vi "switch_curve.vi"(9 "字符串":string, 10 "簇":T23, 11 "配置":T1 {"串口通信UI"."Format" items=["标准帧", "扩展帧"]; "串口通信UI"."Type" items=["数据帧", "远程帧"]; "串口通信UI"."ID" format="0x%x"; "串口通信UI"."Fliter" items=["接收所有类型"=1, "只接收标准帧"=2, "只接收扩展帧"=3]; "串口通信UI"."kBaudRate" items=["5k bps"=1, "10k bps"=2, "20k bps"=3, "40k bps"=4, "50k bps"=5, "80k bps"=6, "100k bps"=7, "125k bps"=8, "200k bps"=9, "250k bps"=10, "400k bps"=11, "500k bps"=12, "666k bps"=13, "800k bps"=14, "1000k bps"=15, "33.33k bps"=16, "66.66k bps"=17, "83.33k bps"=18]; "串口通信UI"."Mode" items=["正常工作", "仅侦听模式", "自测模式（环回）"]; "串口通信UI"."InitFlag" items=["使用界面设置参数"=1]; "串口通信UI"."AccMask" format="%08x"; "串口通信UI"."AccCode" format="%08x"; "串口通信UI"."Channel" items=["通道1", "通道2"]; "串口通信UI"."DevType" items=["USB-CAN"=3, "USB-CAN2"=4]; "安全报警UI"."操作 8" items=["产生报警信息（不发声），等待手动操作", "产生报警信息（发声），等待手动操作", "产生报警信息（不发声），自动刹车", "产生报警信息（发声），自动刹车", "产生报警信息（不发声），立即自动断电，开启泄放电阻", "产生报警信息（发声），立即自动断电，开启泄放电阻"]; "安全报警UI"."操作 7" items=["产生报警信息（不发声），等待手动操作", "产生报警信息（发声），等待手动操作", "产生报警信息（不发声），自动刹车", "产生报警信息（发声），自动刹车", "产生报警信息（不发声），立即自动断电，开启泄放电阻", "产生报警信息（发声），立即自动断电，开启泄放电阻"]; "安全报警UI"."操作 6" items=["产生报警信息（不发声），等待手动操作", "产生报警信息（发声），等待手动操作", "产生报警信息（不发声），自动刹车", "产生报警信息（发声），自动刹车", "产生报警信息（不发声），立即自动断电，开启泄放电阻", "产生报警信息（发声），立即自动断电，开启泄放电阻"]; "安全报警UI"."操作 5" items=["产生报警信息（不发声），等待手动操作", "产生报警信息（发声），等待手动操作", "产生报警信息（不发声），自动刹车", "产生报警信息（发声），自动刹车", "产生报警信息（不发声），立即自动断电，开启泄放电阻", "产生报警信息（发声），立即自动断电，开启泄放电阻"]; "安全报警UI"."操作 4" items=["产生报警信息（不发声），等待手动操作", "产生报警信息（发声），等待手动操作", "产生报警信息（不发声），自动刹车", "产生报警信息（发声），自动刹车", "产生报警信息（不发声），立即自动断电，开启泄放电阻", "产生报警信息（发声），立即自动断电，开启泄放电阻"]; "安全报警UI"."操作 3" items=["产生报警信息（不发声），等待手动操作", "产生报警信息（发声），等待手动操作", "产生报警信息（不发声），自动刹车", "产生报警信息（发声），自动刹车", "产生报警信息（不发声），立即自动断电，开启泄放电阻", "产生报警信息（发声），立即自动断电，开启泄放电阻"]; "安全报警UI"."操作 2" items=["产生报警信息（不发声），等待手动操作", "产生报警信息（发声），等待手动操作", "产生报警信息（不发声），自动刹车", "产生报警信息（发声），自动刹车", "产生报警信息（不发声），立即自动断电，开启泄放电阻", "产生报警信息（发声），立即自动断电，开启泄放电阻"]; "安全报警UI"."操作" items=["产生报警信息（不发声），等待手动操作", "产生报警信息（发声），等待手动操作", "产生报警信息（不发声），自动刹车", "产生报警信息（发声），自动刹车", "产生报警信息（不发声），立即自动断电，开启泄放电阻", "产生报警信息（发声），立即自动断电，开启泄放电阻"]}) -> (3 "配置输出":T1 {"串口通信UI"."Format" items=["标准帧", "扩展帧"]; "串口通信UI"."Type" items=["数据帧", "远程帧"]; "串口通信UI"."ID" format="0x%x"; "串口通信UI"."Fliter" items=["接收所有类型"=1, "只接收标准帧"=2, "只接收扩展帧"=3]; "串口通信UI"."kBaudRate" items=["5k bps"=1, "10k bps"=2, "20k bps"=3, "40k bps"=4, "50k bps"=5, "80k bps"=6, "100k bps"=7, "125k bps"=8, "200k bps"=9, "250k bps"=10, "400k bps"=11, "500k bps"=12, "666k bps"=13, "800k bps"=14, "1000k bps"=15, "33.33k bps"=16, "66.66k bps"=17, "83.33k bps"=18]; "串口通信UI"."Mode" items=["正常工作", "仅侦听模式", "自测模式（环回）"]; "串口通信UI"."InitFlag" items=["使用界面设置参数"=1]; "串口通信UI"."AccMask" format="%08x"; "串口通信UI"."AccCode" format="%08x"; "串口通信UI"."Channel" items=["通道1", "通道2"]; "串口通信UI"."DevType" items=["USB-CAN"=3, "USB-CAN2"=4]; "安全报警UI"."操作 8" items=["产生报警信息（不发声），等待手动操作", "产生报警信息（发声），等待手动操作", "产生报警信息（不发声），自动刹车", "产生报警信息（发声），自动刹车", "产生报警信息（不发声），立即自动断电，开启泄放电阻", "产生报警信息（发声），立即自动断电，开启泄放电阻"]; "安全报警UI"."操作 7" items=["产生报警信息（不发声），等待手动操作", "产生报警信息（发声），等待手动操作", "产生报警信息（不发声），自动刹车", "产生报警信息（发声），自动刹车", "产生报警信息（不发声），立即自动断电，开启泄放电阻", "产生报警信息（发声），立即自动断电，开启泄放电阻"]; "安全报警UI"."操作 6" items=["产生报警信息（不发声），等待手动操作", "产生报警信息（发声），等待手动操作", "产生报警信息（不发声），自动刹车", "产生报警信息（发声），自动刹车", "产生报警信息（不发声），立即自动断电，开启泄放电阻", "产生报警信息（发声），立即自动断电，开启泄放电阻"]; "安全报警UI"."操作 5" items=["产生报警信息（不发声），等待手动操作", "产生报警信息（发声），等待手动操作", "产生报警信息（不发声），自动刹车", "产生报警信息（发声），自动刹车", "产生报警信息（不发声），立即自动断电，开启泄放电阻", "产生报警信息（发声），立即自动断电，开启泄放电阻"]; "安全报警UI"."操作 4" items=["产生报警信息（不发声），等待手动操作", "产生报警信息（发声），等待手动操作", "产生报警信息（不发声），自动刹车", "产生报警信息（发声），自动刹车", "产生报警信息（不发声），立即自动断电，开启泄放电阻", "产生报警信息（发声），立即自动断电，开启泄放电阻"]; "安全报警UI"."操作 3" items=["产生报警信息（不发声），等待手动操作", "产生报警信息（发声），等待手动操作", "产生报警信息（不发声），自动刹车", "产生报警信息（发声），自动刹车", "产生报警信息（不发声），立即自动断电，开启泄放电阻", "产生报警信息（发声），立即自动断电，开启泄放电阻"]; "安全报警UI"."操作 2" items=["产生报警信息（不发声），等待手动操作", "产生报警信息（发声），等待手动操作", "产生报警信息（不发声），自动刹车", "产生报警信息（发声），自动刹车", "产生报警信息（不发声），立即自动断电，开启泄放电阻", "产生报警信息（发声），立即自动断电，开启泄放电阻"]; "安全报警UI"."操作" items=["产生报警信息（不发声），等待手动操作", "产生报警信息（发声），等待手动操作", "产生报警信息（不发声），自动刹车", "产生报警信息（发声），自动刹车", "产生报警信息（不发声），立即自动断电，开启泄放电阻", "产生报警信息（发声），立即自动断电，开启泄放电阻"]})   [LabVIEW 2018, in "UI.lvlib"]
uses:
  UI.lvlib
  Settings/Settings.ctl
  Acquisition/Hardware Configuration.ctl
  Acquisition/Signal Type.ctl
  Logging/Logging Configuration.ctl
  Logging/Logging.lvlib
  Acquisition/Acquisition.lvlib
  Settings/Settings.lvlib
panel:
  # "参数配置文件"
  # "输入数据文件"
  # "加载电机"
  # "负载电机"
  # "注：每次运行实验时销毁现有所有图像"
  # "参数配置文件"
  # "输入数据文件"
  # "加载电机"
  # "负载电机"
  # "注：每次运行实验时销毁现有所有图像"
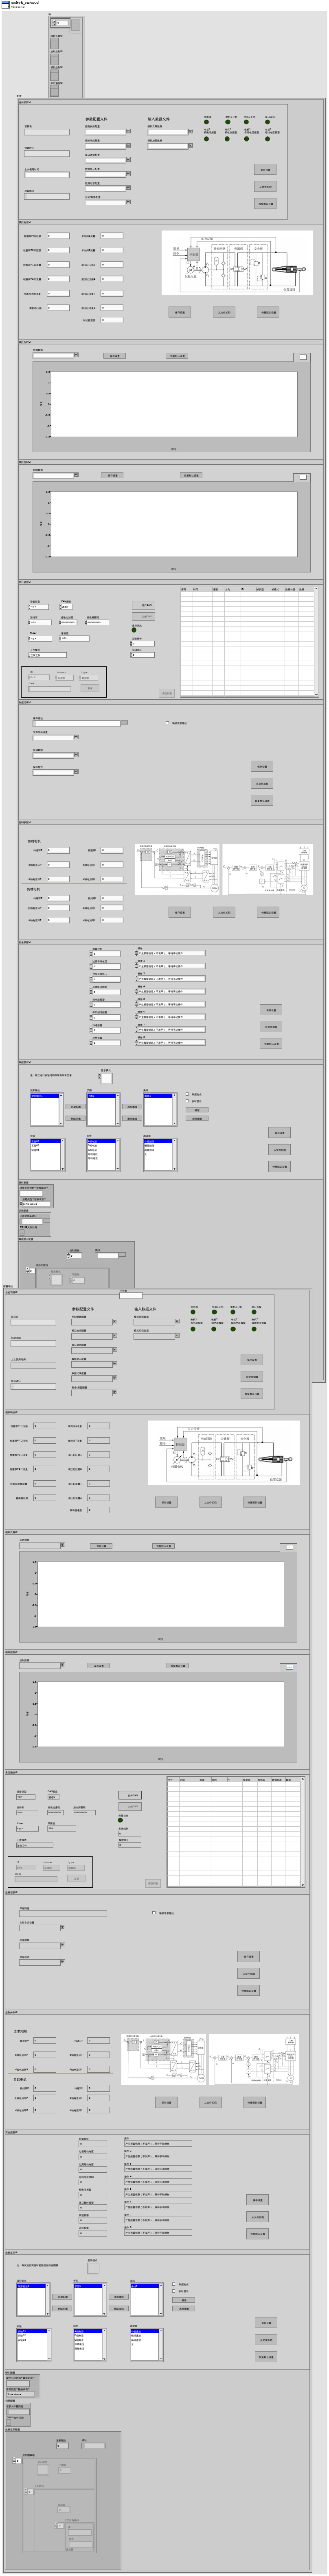
[diagram p1: front panel]
types:
  T1 = typedef "Settings.lvlib/Settings.ctl" = cluster{"当前项目UI":T2, "模拟响应UI":T3, "模拟负载UI":T4, "模拟控制UI":T5, "串口通信UI":T6, "数据记录UI":T12, "控制参数UI":T13, "安全报警UI":T14, "数据显示UI":T15, "硬件配置":T16, "记录配置":T18, "数据显示配置":T19}
  T2 = typedef "控件 5.ctl" = cluster{"控制参数配置":string, "模拟响应配置":string, "串口通信配置":string, "数据显示配置":string, "数据记录配置":string, "安全/报警配置":string, "模拟负载数据":string, "模拟加载数据":string, "总电源":bool, "电机1上电":bool, "电机2上电":bool, "串口连接":bool, "电机1\n相电流报警":bool, "电机2\n相电流报警":bool, "电机1\n母线电压报警":bool, "电机2\n母线电压报警":bool, "保存设置":bool, "从文件加载":bool, "恢复默认设置":bool, "路径":path, "项目路径":path, "项目名":string, "创建时间":string, "上次使用时间":string}
  T3 = typedef "模拟响应UI.ctl" = cluster{"柱塞泵P!口压强":dbl, "柱塞泵P2口压强":dbl, "柱塞泵P1口流量":dbl, "柱塞泵P2口流量":dbl, "柱塞泵泄露流量":dbl, "蓄能器压强":dbl, "单向阀1流量":dbl, "单向阀2流量":dbl, "液压缸压强1":dbl, "液压缸压强2":dbl, "液压缸流量1":dbl, "液压缸流量2":dbl, "做动器速度":dbl, "保存设置":bool, "从文件加载":bool, "恢复默认设置":bool, "路径":path}
  T4 = typedef "控件 9.ctl" = cluster{"负载数据":string, "负载数据 2":waveform(dbl)[], "保存设置":bool, "恢复默认设置":bool}
  T5 = typedef "控件 7.ctl" = cluster{"控制数据":string, "负载数据 2":waveform(dbl)[], "保存设置":bool, "恢复默认设置":bool}
  T6 = typedef "控件 6.ctl" = cluster{"DevType":T7, "Channel":T8, "AccCode":u32, "AccMask":u32, "InitFlag":T9, "Mode":T10, "kBaudRate":u8, "Fliter":T11, "Open":bool, "Close":bool, "连接状态":bool, "SendCnt":u32, "RecvCnt":u32, "Send":bool, "ID":u32, "Data":string, "Type":u8, "Format":u8, "Clear":bool, "list":i32, "路径":path}
  T7 = typedef "ControlCAN.lvlib/DevType.ctl" = u32
  T8 = typedef "ControlCAN.lvlib/CAN Channel.ctl" = u32
  T9 = typedef "ControlCAN.lvlib/InitFlag.ctl" = u32
  T10 = typedef "ControlCAN.lvlib/Mode.ctl" = u8
  T11 = typedef "ControlCAN.lvlib/Fliter.ctl" = u8
  T12 = typedef "控件 3.ctl" = cluster{"保存路径":path, "文件命名设置":string, "存储数据":string, "保存格式":string, "复选框":bool, "保存设置":bool, "从文件加载":bool, "恢复默认设置":bool, "路径":path}
  T13 = typedef "控件 1.ctl" = cluster{"d轴电流环P":dbl, "转速环P":dbl, "q轴电流环P":dbl, "d轴电流环P":dbl, "转矩环P":dbl, "去轴电流环P":dbl, "转速环I":dbl, "q轴电流环I":dbl, "d轴电流环I":dbl, "转矩环I":dbl, "q轴电流环I":dbl, "d轴电流环I":dbl, "保存设置":bool, "从文件加载":bool, "恢复默认设置":bool, "路径":path}
  T14 = typedef "控件 4.ctl" = cluster{"报警扭矩":dbl, "过低母线电压":dbl, "过高母线电压":dbl, "母线电流限制":dbl, "相电流报警":dbl, "串口超时报警":dbl, "转速报警":dbl, "过热报警":dbl, "操作":u16, "操作 2":u16, "操作 3":u16, "操作 4":u16, "操作 5":u16, "操作 6":u16, "操作 7":u16, "操作 8":u16, "保存设置":bool, "从文件加载":bool, "恢复默认设置":bool, "路径":path}
  T15 = typedef "控件 2.ctl" = cluster{"保存设置":bool, "从文件加载":bool, "恢复默认设置":bool, "实验":i32, "波形输出":i32, "组件":i32, "曲线":i32, "滤波器":i32, "删除曲线":bool, "清理图像":bool, "添加曲线":bool, "数据选点":bool, "确定按钮":bool, "实时显示":bool, "子图":i32, "显示模式":u16, "路径":path, "删除图像":bool, "创建新图":bool}
  T16 = typedef "Acquisition.lvlib/Hardware Configuration.ctl" = cluster{"硬件引用句柄<替换此项>":string, "信号类型<替换该项>":T17}
  T17 = typedef "Acquisition.lvlib/Signal Type.ctl" = enum16{"Sine Wave", "Square with Noise"}
  T18 = typedef "Logging.lvlib/Logging Configuration.ctl" = cluster{"记录文件基路径":path, "TDMS文件引用":refnum<k34>}
  T19 = typedef "波形图簇.ctl" = cluster{"波形图数":u32, "波形图数组":T20[], "路径":path}
  T20 = typedef "波形图.ctl" = cluster{"显示模式":u16, "子图数":u32, "子图数组":T21[]}
  T21 = typedef "子图.ctl" = cluster{"子图所有曲线":T22[], "曲线数":u32}
  T22 = typedef "曲线簇.ctl" = cluster{"源":string, "组件":string, "滤波器":string}
  T23 = typedef "引用簇.ctl" = cluster{"数组":refnum<vi>[], "模拟负载UI":refnum<vi>, "波形控制UI":refnum<vi>, "模拟控制UI":refnum<vi>, "串口通信UI":refnum<vi>, "当前项目UI":refnum<vi>, "安全报警UI":refnum<vi>, "数据记录UI":refnum<vi>, "数据显示UI":refnum<vi>, "控制参数UI":refnum<vi>, "模拟响应UI":refnum<vi>, "主选项卡UI":refnum<vi>, "项目管理UI":refnum<vi>, "开始":refnum<vi>, "设置":refnum<vi>, "停止":refnum<vi>, "退出":refnum<vi>}
  T24 = enum8{"Enabled", "Disabled", "Disabled and Grayed Out"}
  T25 = typedef "组件常量.ctl" = string[]
  T26 = typedef "滤波器常量.ctl" = string[]
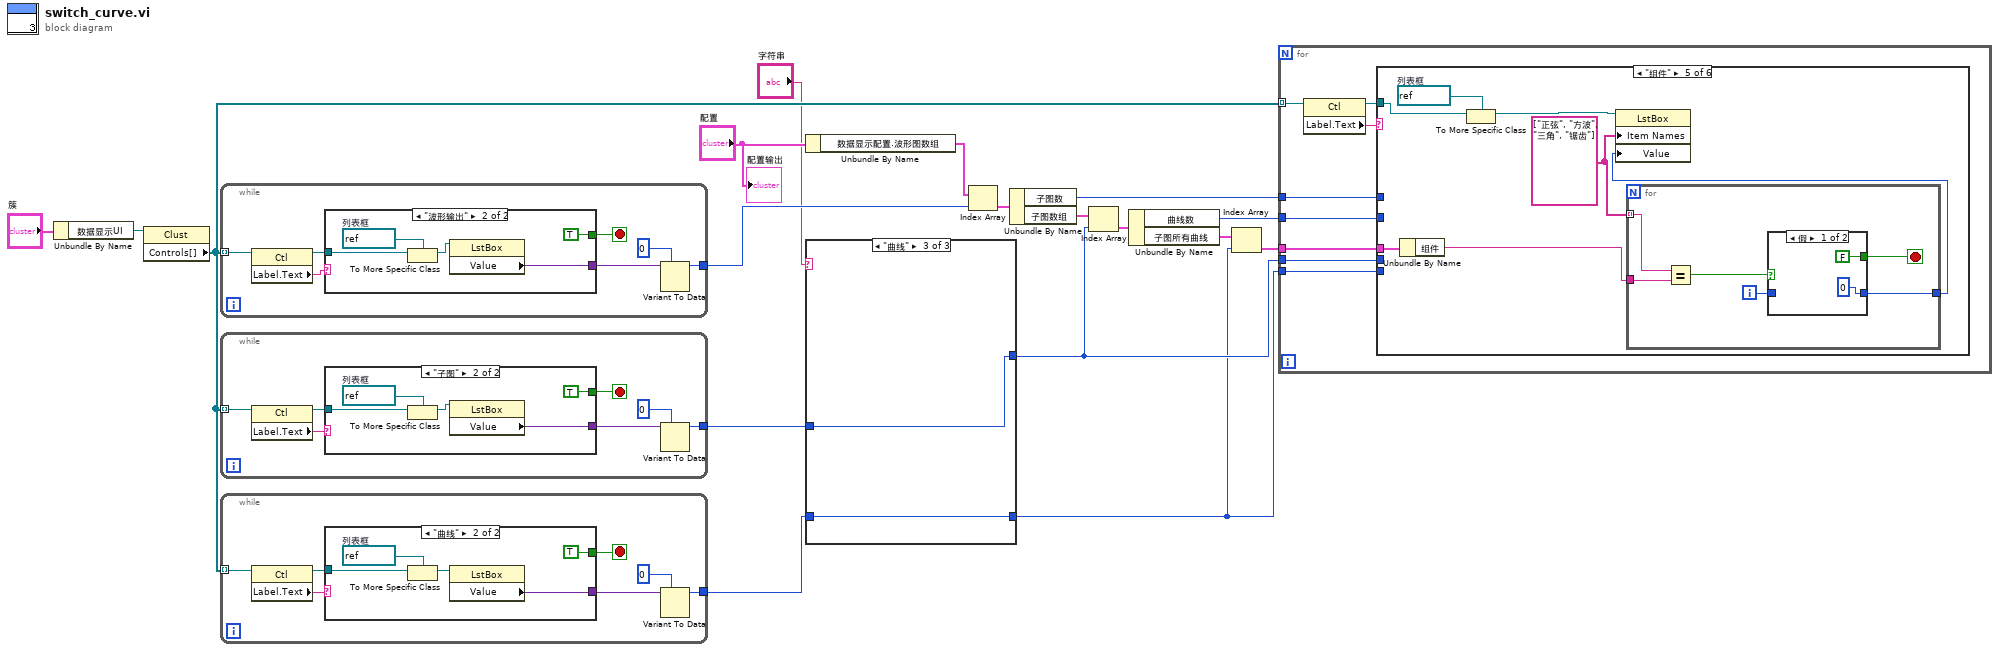
[diagram p0: block diagram]
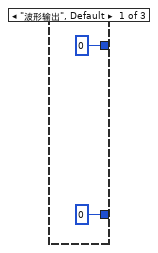
[diagram p2: hidden frame]
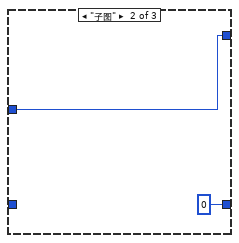
[diagram p3: hidden frame]
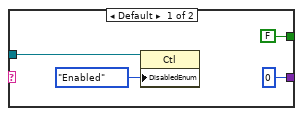
[diagram p4: hidden frame]
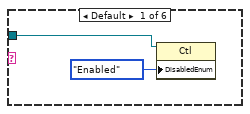
[diagram p5: hidden frame]
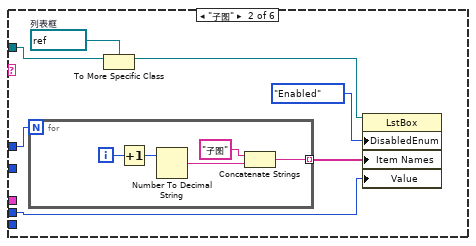
[diagram p6: hidden frame]
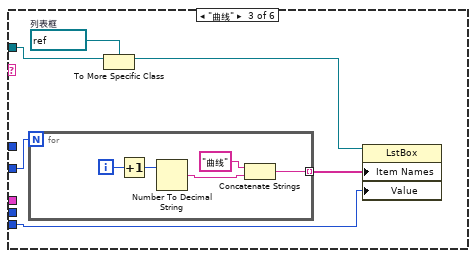
[diagram p7: hidden frame]
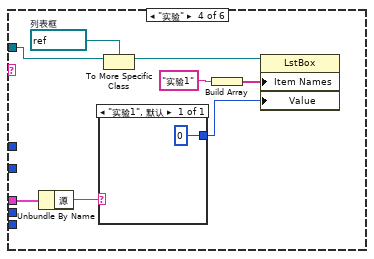
[diagram p8: hidden frame]
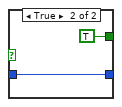
[diagram p9: hidden frame]
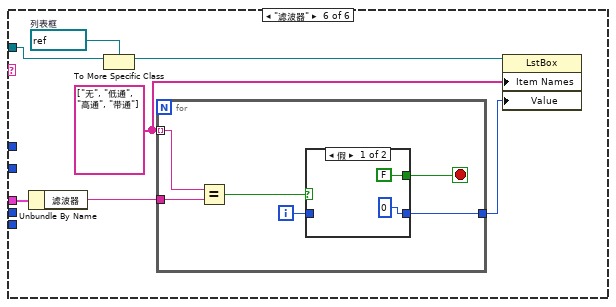
[diagram p10: hidden frame]
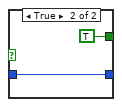
[diagram p11: hidden frame]
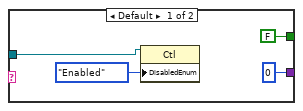
[diagram p12: hidden frame]
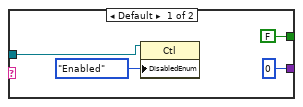
[diagram p13: hidden frame]
diagram:
  n1 = Unbundle By Name("簇") -> ("数据显示UI"=w17:refnum<vi>)
  n2 = property class="Clust"(reference=w17) -> ("Controls[]"=w8:refnum<vi>[])  [unwired: 1 in, 2 out]
  n3 = while {
    tunnel: w8 -> [w25] mode=indexing
    tunnel: [w20] -> w14
    stop <- w22 stop-if-true
    n4 = property class="Ctl"(reference=w25) -> (reference out=w23:refnum<vi>, "Label.Text"=w24:string)  [unwired: 1 in, 1 out]
    n5 = case shown="\"波形输出\"" w24 {
      tunnel: w23 -> [w29 w34]
      tunnel: [0 w30] -> w21
      tunnel: [FALSE TRUE] -> w22
      frame Default {
        n6 = property class="Ctl"(reference=w29, "DisabledEnum"=T24."Enabled" ("禁用")) -> ()  [unwired: 1 in, 2 out]
      }
      frame "波形输出" {
        w33 = refnum<vi> refnum  # 列表框
        n7 = To More Specific Class(target class=w33, reference=w34) -> (specific class reference=w32:refnum<vi>)  [unwired: 1 in, 1 out]
        n8 = property class="LstBox"(reference=w32) -> ("Value"=w30:variant)  [unwired: 1 in, 2 out]
      }
    }
    n9 = Variant To Data(type=0, Variant=w21) -> (data=w20:i32)  [unwired: 1 in, 1 out]
  }
  n10 = while {
    tunnel: w8 -> [w41] mode=indexing
    tunnel: [w36] -> w3
    stop <- w38 stop-if-true
    n11 = property class="Ctl"(reference=w41) -> (reference out=w39:refnum<vi>, "Label.Text"=w40:string)  [unwired: 1 in, 1 out]
    n12 = case shown="\"子图\"" w40 {
      tunnel: w39 -> [w45 w50]
      tunnel: [0 w46] -> w37
      tunnel: [FALSE TRUE] -> w38
      frame Default {
        n13 = property class="Ctl"(reference=w45, "DisabledEnum"=T24."Enabled" ("禁用")) -> ()  [unwired: 1 in, 2 out]
      }
      frame "子图" {
        w49 = refnum<vi> refnum  # 列表框
        n14 = To More Specific Class(target class=w49, reference=w50) -> (specific class reference=w48:refnum<vi>)  [unwired: 1 in, 1 out]
        n15 = property class="LstBox"(reference=w48) -> ("Value"=w46:variant)  [unwired: 1 in, 2 out]
      }
    }
    n16 = Variant To Data(type=0, Variant=w37) -> (data=w36:i32)  [unwired: 1 in, 1 out]
  }
  n17 = while {
    tunnel: w8 -> [w57] mode=indexing
    tunnel: [w52] -> w2
    stop <- w54 stop-if-true
    n18 = property class="Ctl"(reference=w57) -> (reference out=w55:refnum<vi>, "Label.Text"=w56:string)  [unwired: 1 in, 1 out]
    n19 = case shown="\"曲线\"" w56 {
      tunnel: w55 -> [w61 w66]
      tunnel: [0 w62] -> w53
      tunnel: [FALSE TRUE] -> w54
      frame Default {
        n20 = property class="Ctl"(reference=w61, "DisabledEnum"=T24."Enabled" ("禁用")) -> ()  [unwired: 1 in, 2 out]
      }
      frame "曲线" {
        w65 = refnum<vi> refnum  # 列表框
        n21 = To More Specific Class(target class=w65, reference=w66) -> (specific class reference=w64:refnum<vi>)  [unwired: 1 in, 1 out]
        n22 = property class="LstBox"(reference=w64) -> ("Value"=w62:variant)  [unwired: 1 in, 2 out]
      }
    }
    n23 = Variant To Data(type=0, Variant=w53) -> (data=w52:i32)  [unwired: 1 in, 1 out]
  }
  n24 = Unbundle By Name("配置") -> ("数据显示配置.波形图数组"=w15:T20[])
  n25 = case shown="\"曲线\"" "字符串" {
    tunnel: [0 w69 w72] -> w5
    tunnel: [0 0 w71] -> w4
    tunnel: w3 -> [_ w69 w72]
    tunnel: w2 -> [_ _ w71]
    frame "波形输出", Default {
    }
    frame "子图" {
    }
    frame "曲线" {
    }
  }
  n26 = Index Array(array=w15, index=w14) -> (element=w16:T20)
  n27 = Unbundle By Name(w16) -> ("子图数"=w7:u32, "子图数组"=w12:T21[])
  n28 = Index Array(array=w12, index=w5) -> (element=w11:T21)
  n29 = Unbundle By Name(w11) -> ("曲线数"=w1:u32, "子图所有曲线"=w10:T22[])
  n30 = Index Array(array=w10, index=w4) -> (element=w9:T22)
  n31 = for {
    tunnel: w8 -> [w80] mode=indexing
    tunnel: w9 -> [w77]
    tunnel: w4 -> [w76]
    tunnel: w7 -> [w75]
    tunnel: w5 -> [w74]
    tunnel: w1 -> [w73]
    n32 = property class="Ctl"(reference=w80) -> (reference out=w78:refnum<vi>, "Label.Text"=w79:string)  [unwired: 1 in, 1 out]
    n33 = case shown="\"组件\"" w79 {
      tunnel: w78 -> [w82 w85 w96 w113 w121 w138]
      tunnel: w77 -> [_ _ _ w107 w118 w135]
      tunnel: w76 -> [_ _ w100 _ _ _]
      tunnel: w75 -> [_ w84 _ _ _ _]
      tunnel: w74 -> [_ w83 _ _ _ _]
      tunnel: w73 -> [_ _ w95 _ _ _]
      frame Default {
        n34 = property class="Ctl"(reference=w82, "DisabledEnum"=T24."Enabled" ("禁用")) -> ()  [unwired: 1 in, 2 out]
      }
      frame "子图" {
        w88 = refnum<vi> refnum  # 列表框
        n35 = for {
          N: w84 -> [_]
          tunnel: [w92] -> w86 mode=indexing
          i -> [w94]
          n36 = Increment(x=w94) -> (x+1=w90:i32)
          n37 = Number To Decimal String(number=w90) -> (decimal integer string=w91:string)  [unwired: 1 in]
          n38 = Concatenate Strings("子图", w91) -> (w92:string)
        }
        n39 = To More Specific Class(target class=w88, reference=w85) -> (specific class reference=w87:refnum<vi>)  [unwired: 1 in, 1 out]
        n40 = property class="LstBox"(reference=w87, "DisabledEnum"=T24."Enabled" ("禁用"), "Item Names"=w86, "Value"=w83) -> ()  [unwired: 1 in, 2 out]
      }
      frame "曲线" {
        w99 = refnum<vi> refnum  # 列表框
        n41 = for {
          N: w95 -> [_]
          tunnel: [w101] -> w97 mode=indexing
          i -> [w105]
          n42 = Increment(x=w105) -> (x+1=w104:i32)
          n43 = Number To Decimal String(number=w104) -> (decimal integer string=w102:string)  [unwired: 1 in]
          n44 = Concatenate Strings("曲线", w102) -> (w101:string)
        }
        n45 = To More Specific Class(target class=w99, reference=w96) -> (specific class reference=w98:refnum<vi>)  [unwired: 1 in, 1 out]
        n46 = property class="LstBox"(reference=w98, "Item Names"=w97, "Value"=w100) -> ()  [unwired: 1 in, 2 out]
      }
      frame "实验" {
        w112 = refnum<vi> refnum  # 列表框
        n47 = Unbundle By Name(w107) -> ("源"=w108:string)
        n48 = case shown="\"实验1\", 默认" w108 {
          tunnel: [0] -> w106
          frame "实验1", Default {
          }
        }
        n49 = To More Specific Class(target class=w112, reference=w113) -> (specific class reference=w111:refnum<vi>)  [unwired: 1 in, 1 out]
        n50 = Build Array("实验1") -> (w110:string[])
        n51 = property class="LstBox"(reference=w111, "Item Names"=w110, "Value"=w106) -> ()  [unwired: 1 in, 2 out]
      }
      frame "组件" {
        w117 = T25 ["正弦", "方波", "三角", "锯齿"]
        w120 = refnum<vi> refnum  # 列表框
        n52 = Unbundle By Name(w118) -> ("组件"=w116:string)
        n53 = To More Specific Class(target class=w120, reference=w121) -> (specific class reference=w119:refnum<vi>)  [unwired: 1 in, 1 out]
        n54 = for {
          tunnel: w117 -> [w127] mode=indexing
          tunnel: w116 -> [w126]
          tunnel: [w123] -> w115
          i -> [w124]
          stop <- w122 stop-if-true
          n55 = Equal?(x=w127, y=w126) -> (x = y?=w125:bool)
          n56 = case shown="假" w125 {
            tunnel: w124 -> [_ w131]
            tunnel: [0 w131] -> w123
            tunnel: [FALSE TRUE] -> w122
            frame False {
            }
            frame True {
            }
          }
        }
        n57 = property class="LstBox"(reference=w119, "Item Names"=w117, "Value"=w115) -> ()  [unwired: 1 in, 2 out]
      }
      frame "滤波器" {
        w132 = T26 ["无", "低通", "高通", "带通"]
        w137 = refnum<vi> refnum  # 列表框
        n58 = Unbundle By Name(w135) -> ("滤波器"=w134:string)
        n59 = To More Specific Class(target class=w137, reference=w138) -> (specific class reference=w136:refnum<vi>)  [unwired: 1 in, 1 out]
        n60 = for {
          tunnel: w132 -> [w144] mode=indexing
          tunnel: w134 -> [w143]
          tunnel: [w140] -> w133
          i -> [w141]
          stop <- w139 stop-if-true
          n61 = Equal?(x=w144, y=w143) -> (x = y?=w142:bool)
          n62 = case shown="假" w142 {
            tunnel: w141 -> [_ w148]
            tunnel: [0 w148] -> w140
            tunnel: [FALSE TRUE] -> w139
            frame False {
            }
            frame True {
            }
          }
        }
        n63 = property class="LstBox"(reference=w136, "Item Names"=w132, "Value"=w133) -> ()  [unwired: 1 in, 2 out]
      }
    }
  }
  "配置输出" <- "配置"
